vi "FlatToRichgoogle_protobuf_EnumValue.vi"(5 "OutputClusterType":T1, 11 "InputCluster":T4) -> (3 "OutputCluster":T1)   [LabVIEW 2021, in "NI Measurement V2 Client.lvlib"]
uses:
  NI Measurement V2 Client.lvlib
  google_protobuf_EnumValue_Flat.ctl
  google_protobuf_Option_Flat.ctl
  google_protobuf_Any_Flat.ctl
  google_protobuf_EnumValue.ctl
  google_protobuf_Option.ctl
  google_protobuf_Any.ctl
  FlatToRichgoogle_protobuf_Any.vi
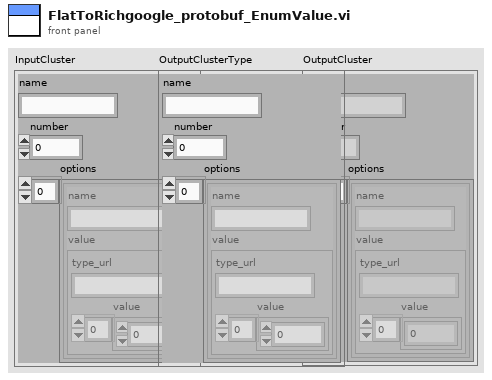
[diagram p1: front panel]
types:
  T1 = typedef "NI Measurement V2 Client.lvlib/google_protobuf_EnumValue.ctl" = cluster{"name":string, "number":i32, "options":T2[]}
  T2 = typedef "NI Measurement V2 Client.lvlib/google_protobuf_Option.ctl" = cluster{"name":string, "value":T3}
  T3 = typedef "NI Measurement V2 Client.lvlib/google_protobuf_Any.ctl" = cluster{"type_url":string, "value":u8[]}
  T4 = typedef "NI Measurement V2 Client.lvlib/google_protobuf_EnumValue_Flat.ctl" = cluster{"name":string, "number":i32, "options":T5[]}
  T5 = typedef "NI Measurement V2 Client.lvlib/google_protobuf_Option_Flat.ctl" = cluster{"name":string, "value":T6}
  T6 = typedef "NI Measurement V2 Client.lvlib/google_protobuf_Any_Flat.ctl" = cluster{"type_url":string, "value":u8[]}
  T7 = typedef "Measurement Service Client V2.lvlib/google_protobuf_Option.ctl" = cluster{"name":string, "value":T8}
  T8 = typedef "Measurement Service Client V2.lvlib/google_protobuf_Any.ctl" = cluster{"type_url":string, "value":u8[]}
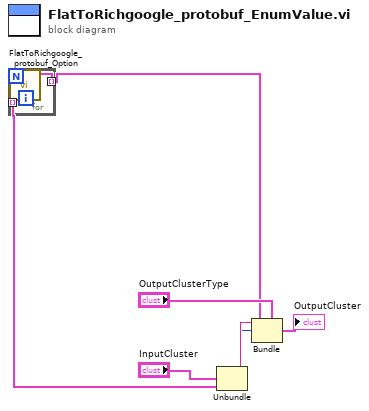
[diagram p0: block diagram]
diagram:
  n1 = Unbundle "Unbundle"("InputCluster") -> ("name"=w4:string, "number"=w3:i32, "options"=w2:T5[])
  n2 = for {
    tunnel: w2 -> [w9] mode=indexing
    tunnel: [w8] -> w1 mode=indexing
    n3 = call "FlatToRichgoogle_protobuf_Option.vi"("InputCluster"=w9) -> ("OutputCluster"=w8:T7)  [unwired: 10 in]
  }
  n4 = Bundle "Bundle"(cluster="OutputClusterType", "name"=w4, "number"=w3, "options"=w1) -> (→"OutputCluster":T1)
